vi "Main.vi"() -> ()   [LabVIEW 2019]
doc: "The myRIO Project template acquires acceleration data from the onboard accelerometer and displays the changes of acceleration values in a waveform chart."
uses:
  <vilib>/myRIO/Common/Instrument Driver Framework/myRIO v1.0/Encoder/typedefs/Encoder Count Direction Enum.ctl
  <vilib>/myRIO/Common/Instrument Driver Framework/myRIO v1.0/Encoder/typedefs/Encoder Signal Mode.ctl
  <vilib>/myRIO/Common/Instrument Driver Framework/myRIO v1.0/Encoder/typedefs/Encoder Channels Enum.ctl
  <vilib>/myRIO/Common/Instrument Driver Framework/Utilities/typedefs/Generic FPGA Reference.ctl
  <vilib>/myRIO/Common/Instrument Driver Framework/Utilities/typedefs/myRIO v1.0 Reference.ctl
  <vilib>/myRIO/Common/Instrument Driver Framework/Utilities/typedefs/Hardware Version Enum.ctl
  <vilib>/myRIO/Common/Instrument Driver Framework/Utilities/typedefs/myRIO Generic Hardware Reference.ctl
  <vilib>/myRIO/Instrument Drivers/Onboard IO/Encoder/typedefs/Encoder Reference.ctl
  <vilib>/myRIO/Instrument Drivers/Onboard IO/Encoder/Encoder.lvlib
  <vilib>/myRIO/Instrument Drivers/Onboard IO/Encoder/vis/Read.vi
  <vilib>/myRIO/Common/Instrument Driver Framework/myRIO v1.0/Encoder/typedefs/Encoder Configuration v1.0.ctl
  <vilib>/userDefined/High Color/nirio_resource_hc.ctl
  <vilib>/myRIO/Common/Instrument Driver Framework/myRIO v1.0/Encoder/vis/myRIO v1.1 Open Encoder.vi
  <vilib>/myRIO/Common/Instrument Driver Framework/myRIO v1.0/Encoder/vis/myRIO v1.0 Configure Encoder.vi
  <vilib>/myRIO/Instrument Drivers/Onboard IO/Encoder/vis/myRIO Encoder Open.xnode
  <vilib>/myRIO/Common/Instrument Driver Framework/Utilities/vis/Is FPGA Ref Available.vi
  <vilib>/myRIO/Express VI/Onboard IO/Encoder/Encoder Express VI.xnode
  <vilib>/myRIO/Instrument Drivers/Utilities/Utilities.lvlib
  <vilib>/Utility/file.llb/Write Delimited Spreadsheet (DBL).vi
panel:
  out "error out":errorcluster
  in  "Stop":bool
  out "Direction 1":enum16{"Counting Up", "Counting Down"}(ring)
  out "Overflow? 1":bool
  in  "Reset":bool
  out "Graph 3":cluster{"ref 1":dbl, "rads":dbl}(graph)
  in  "Freq[Hz]":dbl=1000.0
  out "Direction 2":enum16{"Counting Up", "Counting Down"}(ring)
  out "Overflow? 2":bool
  in  "Reset 2":bool
  out "Duty Cycle out 2":dbl=0.5
  out "Duty Cycle out":dbl=0.5
  out "Graph 2":cluster{dbl, "x2hat":dbl}(graph)
  in  "theta":dbl
  in  "p":dbl
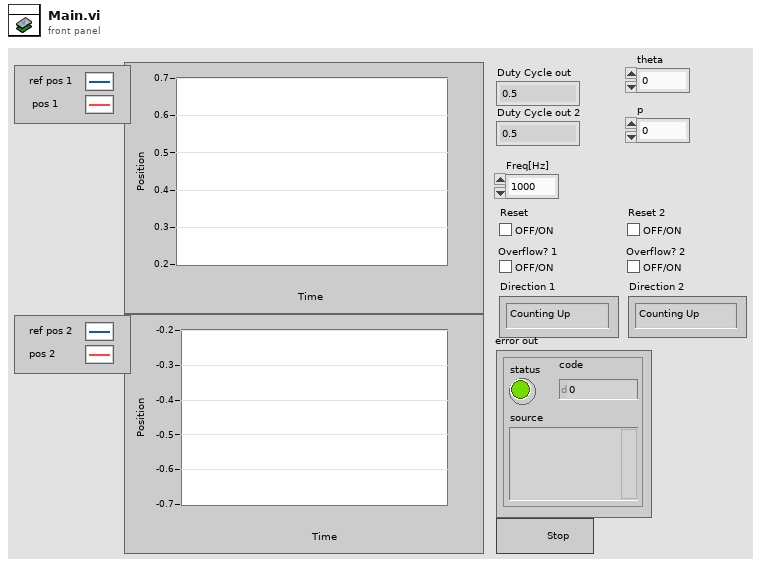
[diagram p1: front panel]
types:
  T1 = typedef "Encoder.lvlib/Encoder Reference.ctl" = cluster{"myRIO Reference":T2, "Encoder Channels Enum":T6}
  T2 = typedef "myRIO Generic Hardware Reference.ctl" = cluster{"myRIO Model":T3, "myRIO Hardware Reference":T4}
  T3 = typedef "Hardware Version Enum.ctl" = enum16{"Unknown", "myRIO-1900", "myRIO-1950", "roboRIO", "NI ELVIS RIO CM", "ELVIS III"}
  T4 = typedef "myRIO v1.0 Reference.ctl" = cluster{"Generic FPGA Reference":T5, "Allow multiple opens":bool}
  T5 = typedef "Generic FPGA Reference.ctl" = refnum<k20>
  T6 = typedef "Encoder Channels Enum.ctl" = enum16{"Not Connected", "C/ENC0", "C/ENC1", "A/ENC", "A/ENC0", "A/ENC1", "A/ENC2", "A/ENC3", "A/ENC4", "A/ENC5", "A/ENC6", "A/ENC7", "A/ENC8", "A/ENC9", "B/ENC", "B/ENC0", "B/ENC1", "B/ENC2", "B/ENC3", "B/ENC4", "B/ENC5", "B/ENC6", "B/ENC7", "B/ENC8", "B/ENC9", "DIO/ENC0", "DIO/ENC1", "DIO/ENC2", "DIO/ENC3", "DIO/ENC4"}
  T7 = typedef "Encoder Signal Mode.ctl" = enum16{"Quadrature phase signal", "Step and direction signal"}
  T8 = typedef "nirio_resource_hc.ctl" = tag
  T9 = typedef "Encoder Count Direction Enum.ctl" = enum16{"Counting Up", "Counting Down"}
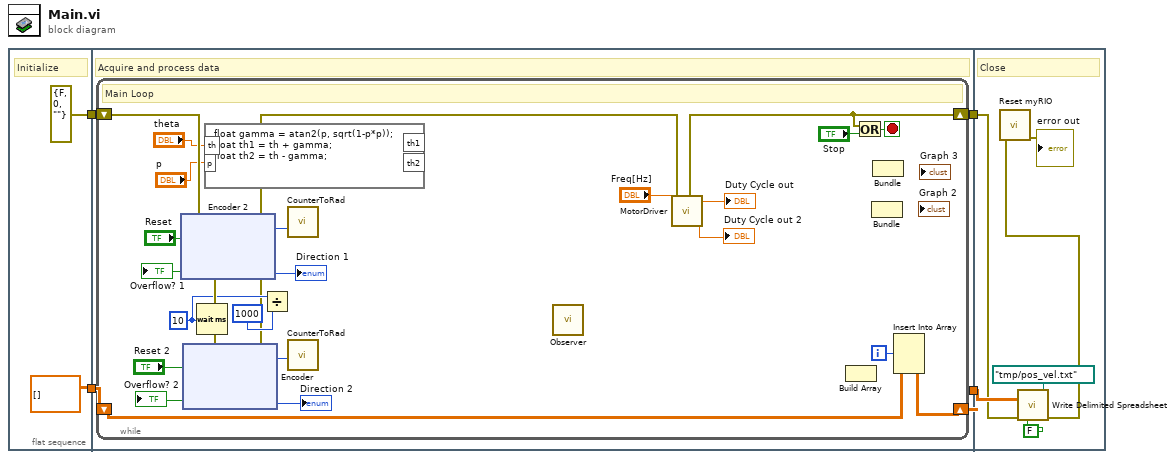
[diagram p0: block diagram]
diagram:
  n1 = flat-sequence {
    tunnel: [errorcluster {"status"=FALSE, "code"=0, "source"=""} ("error in (no error)")] -> w4
    tunnel: [dbl[][] [] ("array")] -> w3
    tunnel: w4 -> [w10]
    tunnel: w3 -> [w9]
    tunnel: [w8] -> w2
    tunnel: [w7] -> w1
    tunnel: w2 -> [w130]
    tunnel: w1 -> [w131]
    frame #0 {
      # "Initialize"
    }
    frame #1 {
      # "Acquire and process data"
      n2 = while {
        shift-right: [w14] -> w8
        shift-left: w10 -> [w27]
        shift-right: [w29] -> w7
        shift-left: w9 -> [w28]
        i -> [w26]
        stop <- w33 stop-if-true
        w20 = u32 10 ("milliseconds to wait")
        # "Main Loop"
        n3 = xnode "Encoder 2"("error in (no error)"=w27, "Reset Counter"="Reset") -> ("error out"=w22:errorcluster, "Counter Value"=w19:i32, "Counter Direction"=→"Direction 1":T9, "Overflow?"=→"Overflow? 1":bool)
        n4 = xnode "Encoder"("error in (no error)"=w22, "Reset Counter"="Reset 2") -> ("error out"=w15:errorcluster, "Counter Value"=w18:i32, "Counter Direction"=→"Direction 2":T9, "Overflow?"=→"Overflow? 2":bool)
        n5 = Wait (ms)(milliseconds to wait=w20) -> ()  [unwired: 1 out]
        n6 = formula code="float gamma = atan2(p, sqrt(1-p*p));\nfloat th1 = th + gamma;\nfloat th2 = th - gamma;"("p"="p", "th"="theta") -> ()  [unwired: 2 out]
        n7 = Divide(x=w20, y=u32 1000) -> ()  [unwired: 1 out]
        n8 = call "CounterToRad.vi"("Counter Value"=w19) -> ()  [unwired: 10 in, 1 out]
        n9 = call "CounterToRad.vi"("Counter Value"=w18) -> ()  [unwired: 10 in, 1 out]
        n10 = call "Observer.vi"() -> ()  [unwired: 11 in, 1 out]
        n11 = call "MotorDriver.vi"("Frequency [Hz]"="Freq[Hz]", "Frequency [Hz] 2"="Freq[Hz]", "error in (no error)"=w15) -> ("Duty Cycle out"=→"Duty Cycle out":dbl, "Duty Cycle out 2"=→"Duty Cycle out 2":dbl, "error out"=w14:errorcluster)  [unwired: 10 in]
        n12 = Build Array() -> ()  [unwired: 2 in, 1 out]
        n13 = Or(x=w14, y="Stop") -> (x .or. y?=w33:bool)
        n14 = Bundle() -> ()  [unwired: 3 in, 1 out]
        n15 = Bundle() -> ()  [unwired: 3 in, 1 out]
        n16 = Insert Into Array(array=w28, index (row)=w26) -> (w29:dbl[][])  [unwired: 2 in]
      }
    }
    frame #2 {
      # "Close"
      n17 = call-poly <vilib>:"Write Delimited Spreadsheet.vi"("file path (dialog if empty)"=path "/tmp/pos_vel.txt", "2D data"=w131, "error in (no error)"=w130, "transpose? (no:F)"=FALSE) -> ("error out"=w129:errorcluster)  [unwired: 10 in, 1 out]
      n18 = call <vilib>:"Reset myRIO.vi"("error in (no error)"=w129) -> ("error out"=→"error out":errorcluster)  [unwired: 10 in]
    }
  }
